vi "Smart Kitchen.vi"() -> ()   [LabVIEW 2022 SP3]
uses:
  <vilib>/DAQmx/read.llb/DAQmx Read (Analog 1D DBL NChan 1Samp).vi
  <vilib>/DAQmx/write.llb/DAQmx Write (Digital Bool 1Line 1Point).vi
  <vilib>/DAQmx/create/channels.llb/DAQmx Create Channel (AI-Voltage-Basic).vi
  <vilib>/DAQmx/create/channels.llb/DAQmx Create Channel (DO-Digital Output).vi
  <vilib>/DAQmx/miscellaneous.llb/DAQmx Fill In Error Info.vi
panel:
  in  "lines 3":tag
  in  "lines 5":tag
  out "min value":dbl
  out "Waveform Chart 3":dbl(graph)
  out "Full":bool
  out "Mid Level":bool
  out "Low Level":bool
  out "Empty":bool
  in  "window":tag
  out "Boolean":bool
  out "element 2":dbl
  in  "for fan":tag
  out "element":dbl
  out "Waveform Chart 2":dbl(graph)
  in  "lines 2":tag
  in  "lines":tag
  out "Waveform Chart":dbl(graph)
  in  "stop":bool
  in  "IR sensor input":tag
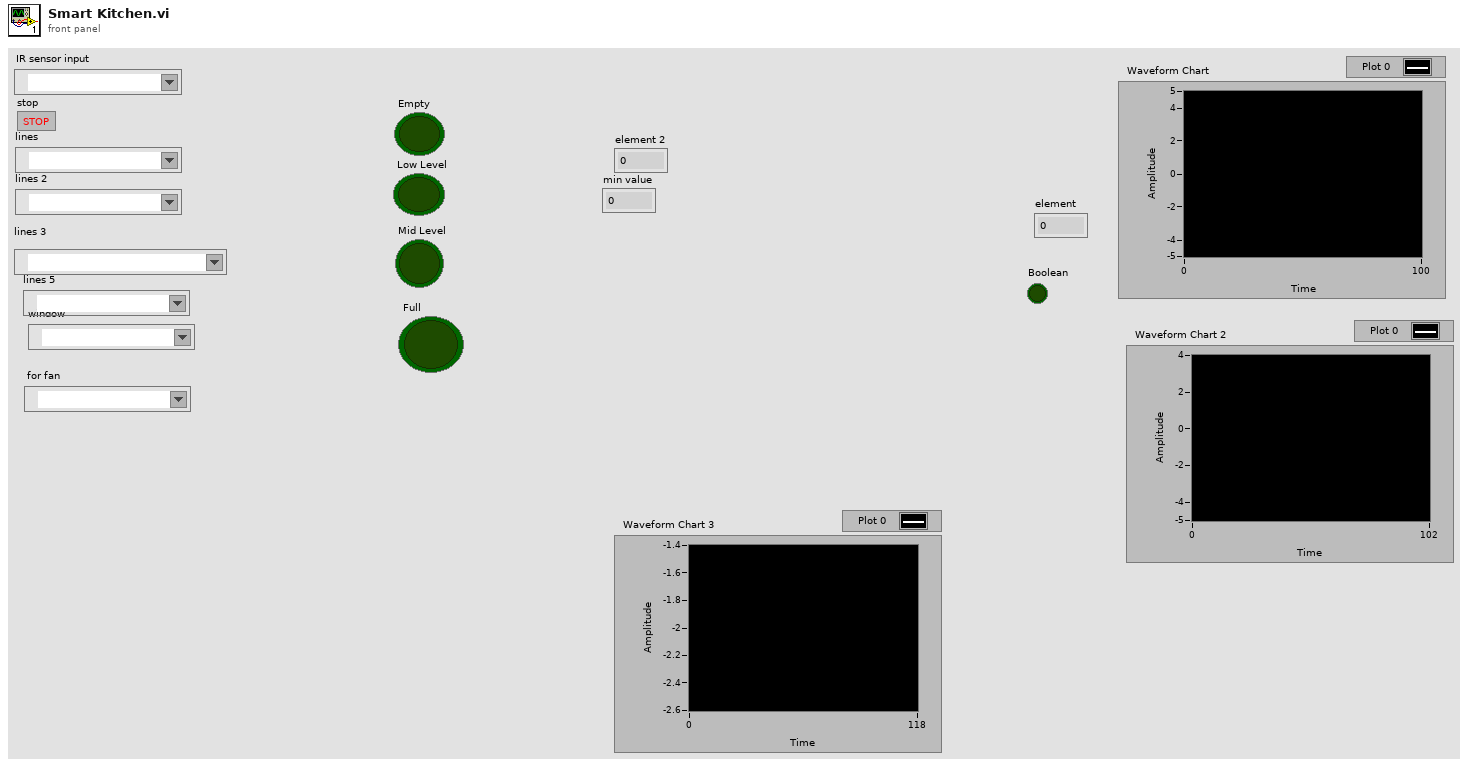
[diagram p1: front panel]
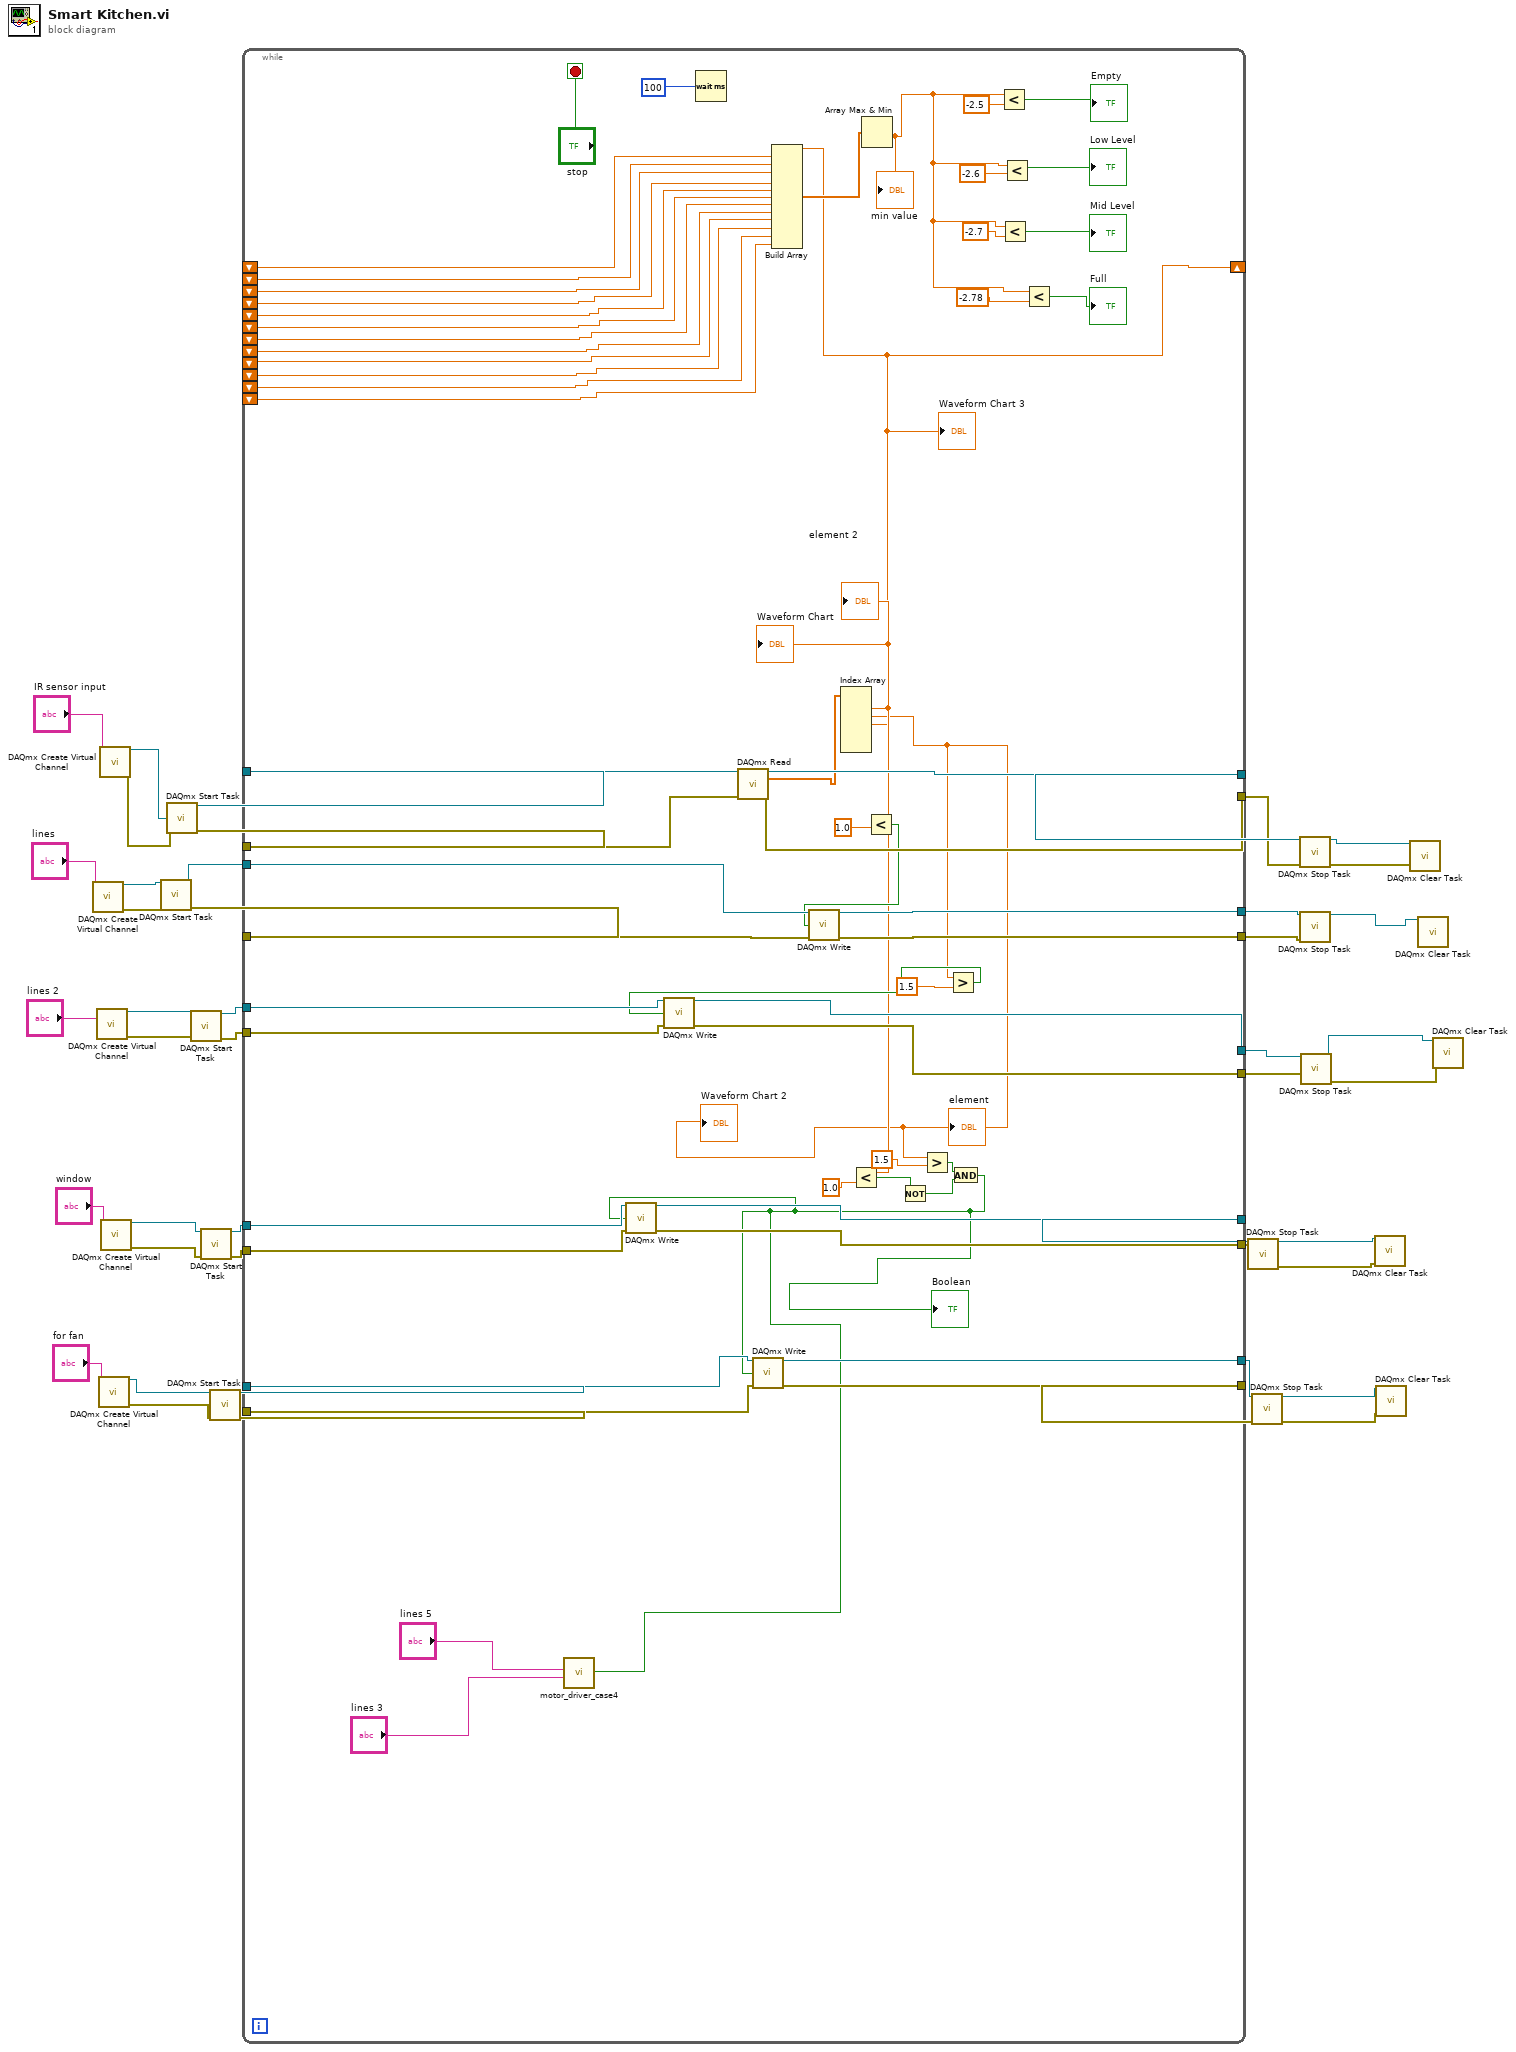
[diagram p0: block diagram]
diagram:
  n1 = call-poly <vilib>:"DAQmx Create Virtual Channel.vi"("lines"="lines") -> ("task out"=w39:refnum<k21>, "error out"=w37:errorcluster)  [unwired: 13 in]
  n2 = call-poly <vilib>:"DAQmx Create Virtual Channel.vi"("lines"="lines 2") -> ("task out"=w27:refnum<k21>, "error out"=w22:errorcluster)  [unwired: 13 in]
  n3 = call-poly <vilib>:"DAQmx Create Virtual Channel.vi"("lines"="for fan") -> ("task out"=w9:refnum<k21>, "error out"=w5:errorcluster)  [unwired: 13 in]
  n4 = call-poly <vilib>:"DAQmx Create Virtual Channel.vi"("physical channels"="IR sensor input") -> ("task out"=w43:refnum<k21>, "error out"=w42:errorcluster)  [unwired: 13 in]
  n5 = call-poly <vilib>:"DAQmx Create Virtual Channel.vi"("lines"="window") -> ("task out"=w18:refnum<k21>, "error out"=w14:errorcluster)  [unwired: 13 in]
  n6 = call <vilib>:"DAQmx Start Task.vi"("task/channels in"=w39, "error in"=w37) -> ("task out"=w32:refnum<k21>, "error out"=w31:errorcluster)  [unwired: 12 in]
  n7 = call <vilib>:"DAQmx Start Task.vi"("task/channels in"=w43, "error in"=w42) -> ("task out"=w36:refnum<k21>, "error out"=w35:errorcluster)  [unwired: 12 in]
  n8 = call <vilib>:"DAQmx Start Task.vi"("task/channels in"=w27, "error in"=w22) -> ("task out"=w26:refnum<k21>, "error out"=w21:errorcluster)  [unwired: 12 in]
  n9 = call <vilib>:"DAQmx Start Task.vi"("task/channels in"=w18, "error in"=w14) -> ("task out"=w17:refnum<k21>, "error out"=w13:errorcluster)  [unwired: 12 in]
  n10 = call <vilib>:"DAQmx Start Task.vi"("task/channels in"=w9, "error in"=w5) -> ("task out"=w8:refnum<k21>, "error out"=w4:errorcluster)  [unwired: 12 in]
  n11 = while {
    tunnel: w36 -> [w104]
    tunnel: w35 -> [w103]
    tunnel: [w102] -> w34
    tunnel: [w101] -> w33
    tunnel: w32 -> [w99]
    tunnel: w31 -> [w98]
    tunnel: [w97] -> w30
    tunnel: [w96] -> w29
    tunnel: w26 -> [w94]
    tunnel: [w93] -> w24
    tunnel: w21 -> [w92]
    tunnel: [w91] -> w20
    tunnel: w17 -> [w87]
    tunnel: [w86] -> w16
    tunnel: w13 -> [w85]
    tunnel: [w84] -> w12
    tunnel: w8 -> [w83]
    tunnel: [w82] -> w7
    tunnel: w4 -> [w81]
    tunnel: [w80] -> w3
    shift-right: [w53] -> _
    shift-left: _ -> [w70]
    shift-left: _ -> [w69]
    shift-left: _ -> [w68]
    shift-left: _ -> [w67]
    shift-left: _ -> [w66]
    shift-left: _ -> [w65]
    shift-left: _ -> [w64]
    shift-left: _ -> [w63]
    shift-left: _ -> [w62]
    shift-left: _ -> [w61]
    shift-left: _ -> [w60]
    shift-left: _ -> [w59]
    stop <- "stop" stop-if-true
    n12 = Wait (ms)(milliseconds to wait=u32 100 ("millisecond timer value")) -> ()  [unwired: 1 out]
    n13 = call-poly <vilib>:"DAQmx Read.vi"("task/channels in"=w104, "error in"=w103) -> ("task out"=w102:refnum<k21>, "data"=w90:dbl[], "error out"=w101:errorcluster)  [unwired: 11 in]
    n14 = Index Array(array=w90) -> (element #1=w76:dbl, element #2=w73:dbl, element #3=w53:dbl)  [unwired: 6 in, 3 out]
    "Waveform Chart" <- w76
    "Waveform Chart 2" <- w73
    "element" <- w73
    "element 2" <- w76
    "Waveform Chart 3" <- w53
    n15 = Build Array(w53, w70, w69, w68, w67, w66, w65, w64, w63, w62, w61, w60, w59) -> (w71:dbl[])
    n16 = Less?(x=w76, y=1.0 ("x")) -> (x < y?=w75:bool)
    n17 = Array Max & Min(array=w71) -> (min value=w47:dbl)  [unwired: 3 out]
    "min value" <- w47
    n18 = Less?(x=w76, y=1.0) -> (x < y?=w78:bool)
    n19 = call-poly <vilib>:"DAQmx Write.vi"("task/channels in"=w99, "data"=w78, "error in"=w98) -> ("task out"=w97:refnum<k21>, "error out"=w96:errorcluster)  [unwired: 10 in, 1 out]
    n20 = Not(x=w75) -> (.not. x?=w74:bool)
    n21 = Greater?(x=w73, y=1.5 ("x")) -> (0:w79:bool)
    n22 = Greater?(x=w73, y=1.5) -> (0:w88:bool)
    n23 = call-poly <vilib>:"DAQmx Write.vi"("task/channels in"=w94, "data"=w88, "error in"=w92) -> ("task out"=w93:refnum<k21>, "error out"=w91:errorcluster)  [unwired: 10 in, 1 out]
    n24 = And(x=w79, y=w74) -> (x .and. y?=w51:bool)
    "Boolean" <- w51
    n25 = call "motor_driver_case4.vi"("Boolean"=w51, "lines 2"="lines 3", "lines"="lines 5") -> ()  [unwired: 9 in]
    n26 = call-poly <vilib>:"DAQmx Write.vi"("task/channels in"=w87, "data"=w51, "error in"=w85) -> ("task out"=w86:refnum<k21>, "error out"=w84:errorcluster)  [unwired: 10 in, 1 out]
    n27 = call-poly <vilib>:"DAQmx Write.vi"("task/channels in"=w83, "data"=w51, "error in"=w81) -> ("task out"=w82:refnum<k21>, "error out"=w80:errorcluster)  [unwired: 10 in, 1 out]
    n28 = Less?(x=w47, y=-2.5) -> (x < y?=→"Empty":bool)
    n29 = Less?(x=w47, y=-2.7) -> (x < y?=→"Mid Level":bool)
    n30 = Less?(x=w47, y=-2.6) -> (x < y?=→"Low Level":bool)
    n31 = Less?(x=w47, y=-2.78) -> (x < y?=→"Full":bool)
  }
  n32 = call <vilib>:"DAQmx Stop Task.vi"("task/channels in"=w16, "error in"=w12) -> ("task out"=w15:refnum<k21>, "error out"=w11:errorcluster)  [unwired: 12 in]
  n33 = call <vilib>:"DAQmx Stop Task.vi"("task/channels in"=w7, "error in"=w3) -> ("task out"=w6:refnum<k21>, "error out"=w2:errorcluster)  [unwired: 12 in]
  n34 = call <vilib>:"DAQmx Stop Task.vi"("task/channels in"=w34, "error in"=w33) -> ("task out"=w40:refnum<k21>, "error out"=w41:errorcluster)  [unwired: 12 in]
  n35 = call <vilib>:"DAQmx Stop Task.vi"("task/channels in"=w30, "error in"=w29) -> ("task out"=w38:refnum<k21>)  [unwired: 12 in, 1 out]
  n36 = call <vilib>:"DAQmx Stop Task.vi"("task/channels in"=w24, "error in"=w20) -> ("task out"=w23:refnum<k21>, "error out"=w19:errorcluster)  [unwired: 12 in]
  n37 = call <vilib>:"DAQmx Clear Task.vi"("task in"=w15, "error in"=w11) -> ()  [unwired: 13 in, 1 out]
  n38 = call <vilib>:"DAQmx Clear Task.vi"("task in"=w6, "error in"=w2) -> ()  [unwired: 13 in, 1 out]
  n39 = call <vilib>:"DAQmx Clear Task.vi"("task in"=w40, "error in"=w41) -> ()  [unwired: 13 in, 1 out]
  n40 = call <vilib>:"DAQmx Clear Task.vi"("task in"=w38) -> ()  [unwired: 14 in, 1 out]
  n41 = call <vilib>:"DAQmx Clear Task.vi"("task in"=w23, "error in"=w19) -> ()  [unwired: 13 in, 1 out]
